vi "Write Subdiagram Labels.vi"(8 "Error In":errorcluster, 11 "DisableStructure In":refnum<vi>) -> (0 "Error Out":errorcluster, 3 "DisableStructure Out":refnum<vi>)   [LabVIEW 2017, in "Eulogy.lvlib"]
uses:
  Eulogy.lvlib
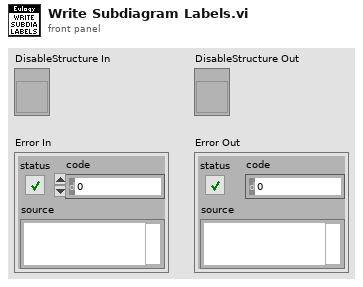
[diagram p1: front panel]
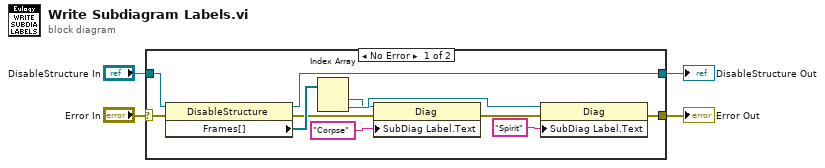
[diagram p0: block diagram]
diagram:
  n1 = case shown="No Error" "Error In" {
    selector: "Error In" -> [w5 w16]
    tunnel: [w15 w16] -> w4
    tunnel: [w14 w17] -> w3
    tunnel: "DisableStructure In" -> [w7 w17]
    frame No Error {
      n2 = property class="DisableStructure"(reference=w7, error in=w5) -> (reference out=w14:refnum<vi>, error out=w6:errorcluster, "Frames[]"=w8:refnum<vi>[])
      n3 = Index Array(array=w8) -> (element #1=w10:refnum<vi>, element #2=w12:refnum<vi>)  [unwired: 2 in]
      n4 = property class="Diag"(reference=w10, error in=w6, "SubDiag Label.Text"="Corpse" ("Subdiagram Label.Text")) -> (error out=w9:errorcluster)  [unwired: 1 out]
      n5 = property class="Diag"(reference=w12, error in=w9, "SubDiag Label.Text"="Spirit" ("Subdiagram Label.Text")) -> (error out=w15:errorcluster)  [unwired: 1 out]
    }
    frame Error {
    }
  }
  "Error Out" <- w4
  "DisableStructure Out" <- w3
